vi "p6100_general.vi"   [LabVIEW 2011]
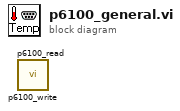
[diagram p0: block diagram]
diagram:
  n1 = call "p6100_write.vi"() -> ()  [unwired: 5 in, 3 out]
  n2 = call "p6100_read.vi"() -> ()  [unwired: 5 in, 3 out]
